vi "LVUseDLL.vi"() -> ()   [LabVIEW 2020]
uses:
  CtoLV.dll
panel:
  out "array_5":i16[][](array[numeric])
  out "Output_Cluster":T1 {"Array Constant" format="%.2f"; "?" format="%.2f"}
  in  "NumberofBools":i32=5
  out "Boolean Array":bool[](array[boolean])
  in  "NumberofStrings":i32=3
  out "StringArray":string[](array[string])
  out "string_out3":string
  in  "String Size":i32=6
  out "string_out2":string
  out "string_out1":string
  in  "string_in":string="hello"
  out "array_5":i16[][](array[numeric])
  in  "cols":i32=3
  in  "rows":i32=2
  out "array_4":dbl[][](array[numeric]) format="%.2f"
  out "array_3":dbl[](array[numeric]) format="%.2f"
  in  "size":i32=5
  out "array_out2":dbl[](array[numeric]) format="%.2f"
  out "array_out1":dbl[](array[numeric]) format="%.2f"
  # "These two examples modify contents of an array using two different methods"
  # "These two example modify the contents of a LV string"
  # "passes string as char*"
  # "Modifies contents of \narray using double*"
  # "passes string as LV structure"
  # "Modifies contents of array \nusing LV structure"
  # "Dynamically allocates space for string"
  # "Dynamically Allocates array"
  # "Dynamically allocates array of strings"
  # "These two examples modify the contents of a 2-D array."
  # "Passed as LV structure"
  # "Passed as double*"
  # "Dynamically allocates array of Booleans"
  # "Dynamically creates a 2-D array and fills it"
  # "This example illustrates how to pass various LabVIEW data types to C code and how to \nhave the C code either modify the contents of the LabVIEW variables or dynamically \nallocate space in LabVIEW for new data and send it back to LabVIEW.  The C code is \nincluded which illustrates how to use some LabVIEW memory manager functions.  For a \nmore detailed description of how LabVIEW stores different types of data in memory,"
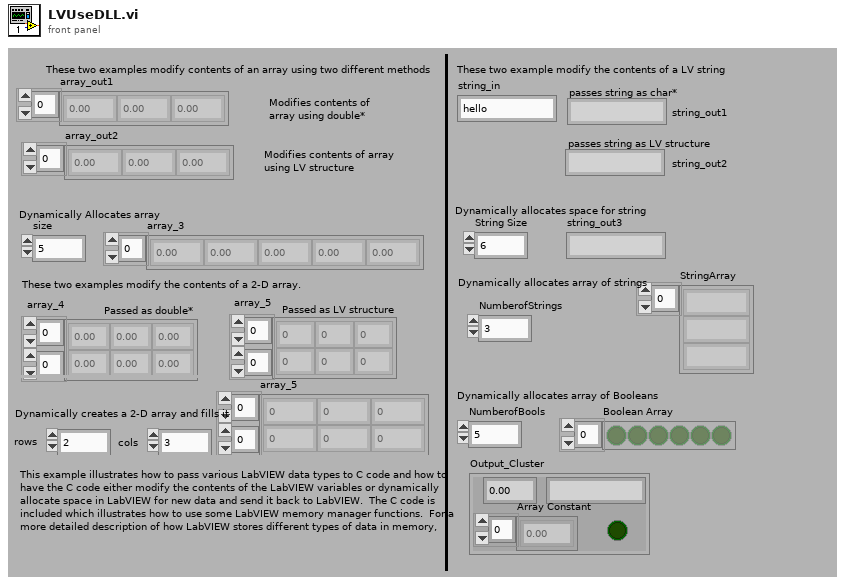
[diagram p1: front panel]
types:
  T1 = cluster{dbl, string, "Array Constant":dbl[], bool}
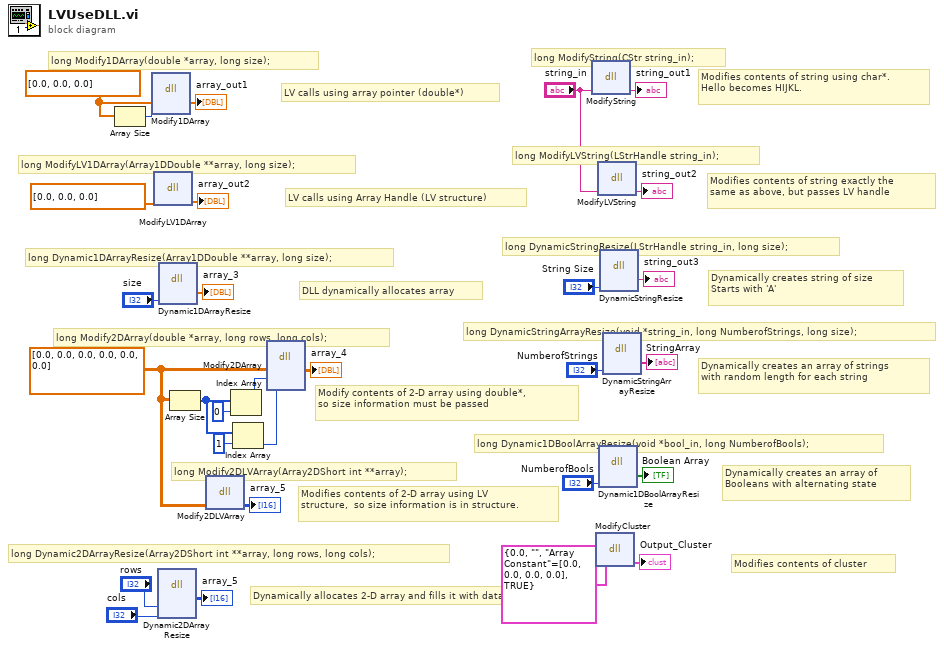
[diagram p0: block diagram]
diagram:
  w2 = dbl[][] [[0.0, 0.0, 0.0], [0.0, 0.0, 0.0]] ("Array Constant")
  w28 = dbl[] [0.0, 0.0, 0.0] ("Array Constant")
  # "Modifies contents of 2-D array using LV \nstructure,  so size information is in structure."
  # "long Modify2DLVArray(Array2DShort int **array);"
  # "Modifies contents of cluster"
  # "Dynamically creates an array of \nBooleans with alternating state"
  # "long Dynamic1DBoolArrayResize(void *bool_in, long NumberofBools);"
  # "Dynamically creates an array of strings \nwith random length for each string"
  # "long DynamicStringArrayResize(void *string_in, long NumberofStrings, long size);"
  # "Dynamically creates string of size\nStarts with 'A'"
  # "long DynamicStringResize(LStrHandle string_in, long size);"
  # "Modifies contents of string exactly the \nsame as above, but passes LV handle"
  # "long ModifyLVString(LStrHandle string_in);"
  # "Modifies contents of string using char*.\nHello becomes HIJKL."
  # "long ModifyString(CStr string_in);"
  # "Dynamically allocates 2-D array and fills it with data"
  # "long Dynamic2DArrayResize(Array2DShort int **array, long rows, long cols);"
  # "Modify contents of 2-D array using double*, \nso size information must be passed"
  # "long Modify2DArray(double *array, long rows, long cols);"
  # "DLL dynamically allocates array"
  # "long Dynamic1DArrayResize(Array1DDouble **array, long size);"
  # "LV calls using Array Handle (LV structure)"
  # "LV calls using array pointer (double*)"
  # "long ModifyLV1DArray(Array1DDouble **array, long size);"
  # "long Modify1DArray(double *array, long size);"
  n1 = Array Size(array=w28) -> (size(s)=w29:i32)
  n2 = dll-call lib="C:/WINNT/Profiles/bbuchana/Desktop/CtoLV.dll" fn="Modify1DArray"("array"=w28, "size"=w29) -> ("array"=→"array_out1":dbl[])  [unwired: 5 in, 2 out]
  n3 = dll-call lib="C:/WINNT/Profiles/bbuchana/Desktop/CtoLV.dll" fn="ModifyLV1DArray"("array"=dbl[] [0.0, 0.0, 0.0] ("Array Constant")) -> ("array"=→"array_out2":dbl[])  [unwired: 4 in, 2 out]
  n4 = dll-call lib="C:/WINNT/Profiles/bbuchana/Desktop/CtoLV.dll" fn="Dynamic2DArrayResize"("rows"="rows", "cols"="cols") -> ("array"=→"array_5":i16[][])  [unwired: 7 in, 2 out]
  n5 = dll-call lib="C:/WINNT/Profiles/bbuchana/Desktop/CtoLV.dll" fn="Dynamic1DArrayResize"("size"="size") -> ("array"=→"array_3":dbl[])  [unwired: 6 in, 2 out]
  n6 = Array Size(array=w2) -> (size(s)=w20:i32[])
  n7 = dll-call lib="C:/WINNT/Profiles/bbuchana/Desktop/CtoLV.dll" fn="Modify2DLVArray"("array"=w2) -> ("array"=→"array_5":i16[][])  [unwired: 4 in, 2 out]
  n8 = Index Array(array=w20, index=0) -> (element=w19:i32)
  n9 = Index Array(array=w20, index=1) -> (element=w18:i32)
  n10 = dll-call lib="C:/WINNT/Profiles/bbuchana/Desktop/CtoLV.dll" fn="Modify2DArray"("array"=w2, "rows"=w19, "cols"=w18) -> ("array"=→"array_4":dbl[][])  [unwired: 6 in, 2 out]
  n11 = dll-call lib="C:/WINNT/Profiles/bbuchana/Desktop/CtoLV.dll" fn="ModifyString"("string_in"="string_in") -> ("string_in"=→"string_out1":string)  [unwired: 4 in, 2 out]
  n12 = dll-call lib="C:/WINNT/Profiles/bbuchana/Desktop/CtoLV.dll" fn="ModifyCluster"(T1 {0.0, "", "Array Constant"=[0.0, 0.0, 0.0, 0.0], TRUE}) -> (→"Output_Cluster":T1)  [unwired: 4 in, 2 out]
  n13 = dll-call lib="C:/WINNT/Profiles/bbuchana/Desktop/CtoLV.dll" fn="ModifyLVString"("string_in"="string_in") -> ("string_in"=→"string_out2":string)  [unwired: 4 in, 2 out]
  n14 = dll-call lib="C:/WINNT/Profiles/bbuchana/Desktop/CtoLV.dll" fn="Dynamic1DBoolArrayResize"("NumberofBools"="NumberofBools") -> ("Boolean Array"=→"Boolean Array":bool[])  [unwired: 6 in, 2 out]
  n15 = dll-call lib="C:/WINNT/Profiles/bbuchana/Desktop/CtoLV.dll" fn="DynamicStringResize"("size"="String Size") -> ("string_in"=→"string_out3":string)  [unwired: 6 in, 2 out]
  n16 = dll-call lib="C:/WINNT/Profiles/bbuchana/Desktop/CtoLV.dll" fn="DynamicStringArrayResize"("NumberofStrings"="NumberofStrings") -> ("StringArray"=→"StringArray":string[])  [unwired: 6 in, 2 out]
